vi "GetExperimentPaths.vi"(0 "MeasureConfig":T1={"Bead locations"=[{"X"=0, "Y"=0}], "ROI"=200, "Experiment base path"=path "", "Image output subdir"="images", "Output mode"=enum."None", "Traces output subdir"="traces", "QTrk Settings"={"Image width"=150, "Image height"=150, "Number of threads (CPU based)"=-1, "CUDA Device"=-2, "COM Background correction factor"=0.0, "ZLUT MinRadius"=8.0, "ZLUT Radial sample density"=5.0, "ZLUT Angular sample density"=2.0, "ZLUT ROI Coverage"=0.7, "QI Iterations"=1, "QI MinRadius"=2.0, "QI Radial sample density"=5.0, "QI Angular sample density"=2.0, "QI ROI Coverage"=0.7, "QI Angular Step \nIteration Factor"=0.8, "XCOR Profile Length"=1, "XCOR Profile Width"=128, "XCOR Iterations"=32, "Gaussian 2D Fit Iterations"=2, "Gaussian 2D Sigma (pixels)"=3.0}, "Tracking Config"={"Number of steps"=0, "ZLUT stepsize (um)"=0.0, "Z correction factor"=0.0, "Start piezo Z (um)"=0.0, "Pixel size (nm)"=0.0, "2D Localization Type"=enum."Quadrant Interpolation", "Z Command (None)"=enum."Nothing", "Z Piezo scale"=FALSE}, "Experiment Name"="", "Program"={"Commands"=[], "Motor Axis accuracy conditions"={"Magnet Z"=0.0, "Magnet rotation"=0.0, "Camera"={"X"=0.0, "Y"=0.0}, "Piezo XY"={"X"=0.0, "Y"=0.0}, "Piezo Z"=0.0}, "Axis flags"={"Magnet Z"=FALSE, "Magnet rotation"=FALSE, "Camera"={"X"=FALSE, "Y"=FALSE}, "Piezo XY"={"X"=FALSE, "Y"=FALSE}, "Piezo Z"=FALSE}}, "ZLUT"=[], "Camera settings"={"Framerate (Hz)"=60, "Exposure time (us)"=5000, "Image size"={"Width"=1280, "Height"=1024}, "Number of buffers"=30}, "Experiment Script"="", "Max frames in memory"=2, "Save traces as binary"=FALSE, "Pixel Calibration Gain Image"="camera_calib_gain.bin", "Pixel Calibration Offset Image"="camera_calib_gain.bin", "Use pixel calibration images"=FALSE, "Internal camera settings"=""} {"QTrk Settings"."QI ROI Coverage" format="%_2g"; "QTrk Settings"."QI MinRadius" format="%.2f"; "QTrk Settings"."QI Angular sample density" format="%.3f"; "QTrk Settings"."QI Radial sample density" format="%.2f"; "QTrk Settings"."ZLUT Radial sample density" format="%.2f"; "QTrk Settings"."ZLUT MinRadius" format="%.2f"}) -> (3 "[base]\\traces\\[expname]_motors.txt":path, 4 "[base]\\images\\[expname]\\":path, 6 "[base]\\traces\\":path, 8 "[base]\\traces\\[expname]_sections.txt":path, 10 "[base]\\beadlist.txt":path, 12 "[base]\\[expname]_script.txt":path, 13 "[base]\\[expname].radialzlut":path, 14 "[base]\\traces\\[expname].txt/bin":path, 15 "[base]\\traces\\[expname]_info.txt":path)   [LabVIEW 2011]
uses:
  Typedefs/MeasureConfigType.ctl
  Typedefs/MeasureConfigOutputMode.ctl
  qtrk/QTrk.llb/QTrkSettings.ctl
  Typedefs/TrackingConfigType.ctl
  qtrk/QTrk.llb/QTrkLocalizationType.ctl
  qtrk/QTrk.llb/QTrkZCommandType.ctl
  ExperimentProgram/ExperimentProgramType.ctl
  ExperimentProgram/ExProgCommandType.ctl
  ExperimentProgram/ExProgCommandEnumType.ctl
  Motors/MotorAxisEnum.ctl
  Motors/MotorPosType.ctl
  Typedefs/XYf.ctl
  Motors/MotorPosFlagsType.ctl
  Camera/GenericCameraConfigType.ctl
panel:
  # "(used for commands with string parameters)"
  # "-2: Use all devices\n-1: Use best device"
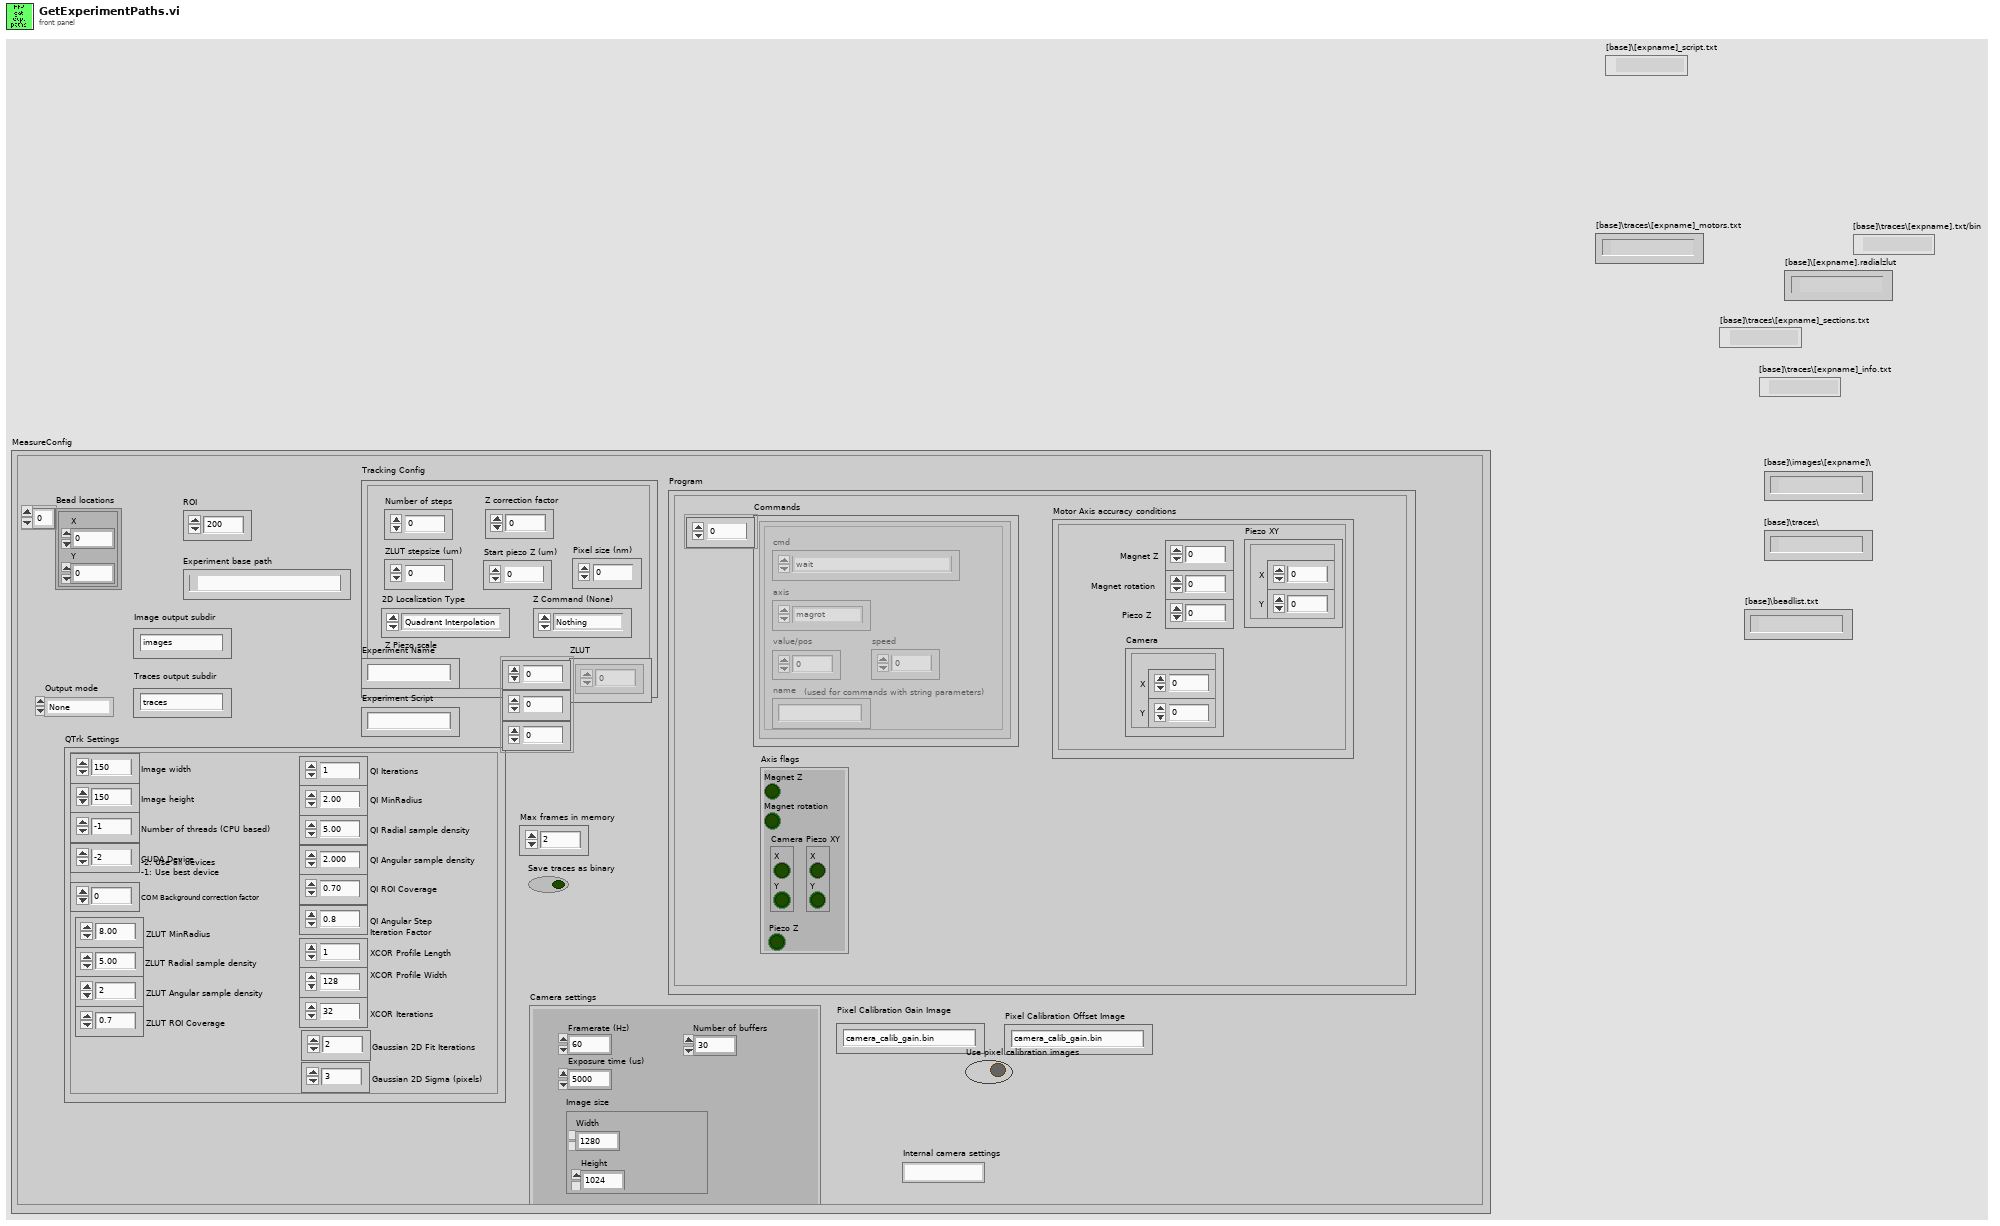
[diagram p1: front panel]
types:
  T1 = typedef "MeasureConfigType.ctl" = cluster{"Bead locations":cluster{"X":i32, "Y":i32}[], "ROI":i32, "Experiment base path":path, "Image output subdir":string, "Output mode":T2, "Traces output subdir":string, "QTrk Settings":T3, "Tracking Config":T4, "Experiment Name":string, "Program":T7, "ZLUT":sgl[][][], "Camera settings":T14, "Experiment Script":string, "Max frames in memory":i32, "Save traces as binary":bool, "Pixel Calibration Gain Image":string, "Pixel Calibration Offset Image":string, "Use pixel calibration images":bool, "Internal camera settings":string}
  T2 = typedef "MeasureConfigOutputMode.ctl" = enum16{"None", "Track", "SaveImages"}
  T3 = typedef "QTrkSettings.ctl" = cluster{"Image width":i32, "Image height":i32, "Number of threads (CPU based)":i32, "CUDA Device":i32, "COM Background correction factor":sgl, "ZLUT MinRadius":sgl, "ZLUT Radial sample density":sgl, "ZLUT Angular sample density":sgl, "ZLUT ROI Coverage":sgl, "QI Iterations":i32, "QI MinRadius":sgl, "QI Radial sample density":sgl, "QI Angular sample density":sgl, "QI ROI Coverage":sgl, "QI Angular Step \nIteration Factor":sgl, "XCOR Profile Length":i32, "XCOR Profile Width":i32, "XCOR Iterations":i32, "Gaussian 2D Fit Iterations":i32, "Gaussian 2D Sigma (pixels)":sgl}
  T4 = typedef "TrackingConfigType.ctl" = cluster{"Number of steps":i32, "ZLUT stepsize (um)":sgl, "Z correction factor":sgl, "Start piezo Z (um)":sgl, "Pixel size (nm)":sgl, "2D Localization Type":T5, "Z Command (None)":T6, "Z Piezo scale":bool}
  T5 = typedef "QTrkLocalizationType.ctl" = enum16{"Center-of-Mass", "1D Cross-Correlation", "Quadrant Interpolation", "Gaussian 2D MLE", "QI + ZLUTAlign", "ZLUTAlign"}
  T6 = typedef "QTrkZCommandType.ctl" = enum16{"Nothing", "ComputeZ", "BuildRadialZLUT", "BuildImageZLUT", "RadialZLUT+ImageZLUT"}
  T7 = typedef "ExperimentProgramType.ctl" = cluster{"Commands":T8[], "Motor Axis accuracy conditions":T11, "Axis flags":T13}
  T8 = typedef "ExProgCommandType.ctl" = cluster{"cmd":T9, "axis":T10, "value/pos":dbl, "speed":dbl, "name":string}
  T9 = typedef "ExProgCommandEnumType.ctl" = enum16{"wait", "move", "acquire", "idle", "rmove", "when", "section", "stop"}
  T10 = typedef "MotorAxisEnum.ctl" = enum16{"no axis", "magrot", "magpos", "px", "py", "pz", "camx", "camy"}
  T11 = typedef "MotorPosType.ctl" = cluster{"Magnet Z":dbl, "Magnet rotation":dbl, "Camera":T12, "Piezo XY":T12, "Piezo Z":dbl}
  T12 = typedef "XYf.ctl" = cluster{"X":sgl, "Y":sgl}
  T13 = typedef "MotorPosFlagsType.ctl" = cluster{"Magnet Z":bool, "Magnet rotation":bool, "Camera":cluster{"X":bool, "Y":bool}, "Piezo XY":cluster{"X":bool, "Y":bool}, "Piezo Z":bool}
  T14 = typedef "GenericCameraConfigType.ctl" = cluster{"Framerate (Hz)":i32, "Exposure time (us)":i32, "Image size":cluster{"Width":i32, "Height":i32}, "Number of buffers":i32}
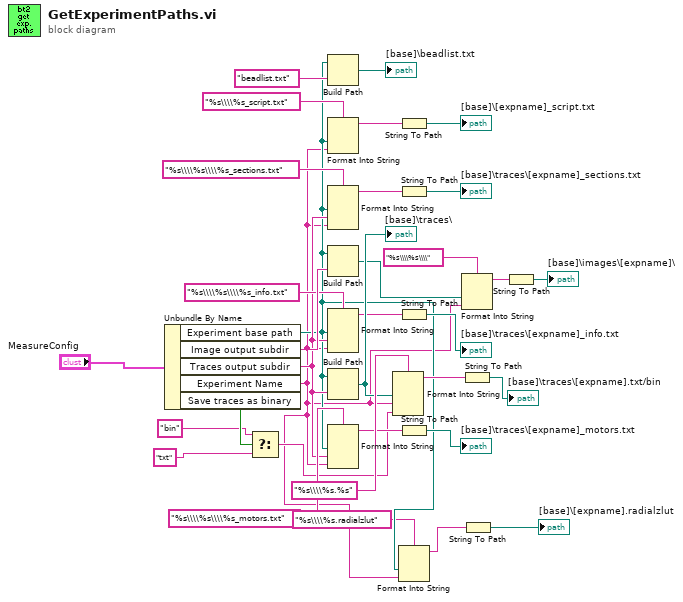
[diagram p0: block diagram]
diagram:
  n1 = Unbundle By Name("MeasureConfig") -> ("Experiment base path"=w3:path, "Image output subdir"=w33:string, "Traces output subdir"=w12:string, "Experiment Name"=w2:string, "Save traces as binary"=w9:bool)
  n2 = Select(t="bin" ("format string"), s=w9, f="txt" ("format string")) -> (s? t:f=w6:string)
  n3 = Build Path(base path=w3, name or relative path="beadlist.txt") -> (appended path=→"[base]\\beadlist.txt":path)
  n4 = Format Into String(format string="%s\\\\%s_script.txt", w3, w2) -> (resulting string=w15:string)  [unwired: 2 in, 1 out]
  n5 = Format Into String(format string="%s\\\\%s\\\\%s_sections.txt", w3, w12, w2) -> (resulting string=w11:string)  [unwired: 2 in, 1 out]
  n6 = Build Path(base path=w3, name or relative path=w33) -> (appended path=w25:path)
  n7 = Format Into String(format string="%s\\\\%s\\\\%s_info.txt", w3, w12, w2) -> (resulting string=w21:string)  [unwired: 2 in, 1 out]
  n8 = Build Path(base path=w3, name or relative path=w12) -> (appended path=w29:path)
  "[base]\\traces\\" <- w29
  n9 = Format Into String(format string="%s\\\\%s\\\\%s_motors.txt", w3, w12, w2) -> (resulting string=w18:string)  [unwired: 2 in, 1 out]
  n10 = Format Into String(format string="%s\\\\%s.%s", w29, w2, w6) -> (resulting string=w28:string)  [unwired: 2 in, 1 out]
  n11 = String To Path(string=w15) -> (path=→"[base]\\[expname]_script.txt":path)
  n12 = String To Path(string=w11) -> (path=→"[base]\\traces\\[expname]_sections.txt":path)
  n13 = String To Path(string=w21) -> (path=→"[base]\\traces\\[expname]_info.txt":path)
  n14 = String To Path(string=w18) -> (path=→"[base]\\traces\\[expname]_motors.txt":path)
  n15 = Format Into String(format string="%s\\\\%s.radialzlut", w3, w2) -> (resulting string=w5:string)  [unwired: 2 in, 1 out]
  n16 = Format Into String(format string="%s\\\\%s\\\\", w25, w2) -> (resulting string=w23:string)  [unwired: 2 in, 1 out]
  n17 = String To Path(string=w28) -> (path=→"[base]\\traces\\[expname].txt/bin":path)
  n18 = String To Path(string=w5) -> (path=→"[base]\\[expname].radialzlut":path)
  n19 = String To Path(string=w23) -> (path=→"[base]\\images\\[expname]\\":path)
